vi "BP_outputLayer.vi"(0 "Target_outX":dbl[](array[numeric]), 1 "Out_hx":dbl[](array[numeric]), 2 "Out_outX":dbl[](array[numeric]), 3 "Learning rate":dbl, 4 "Weights_outX_IN":dbl[][](array[numeric])) -> (5 "Weights_outX_OUT":dbl[][](array[numeric]))   [LabVIEW 2016]
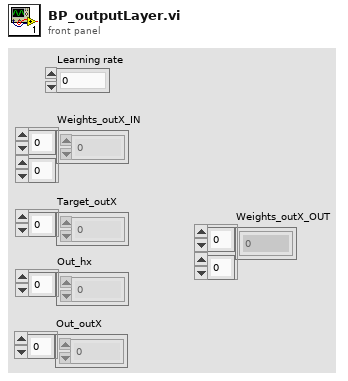
[diagram p1: front panel]
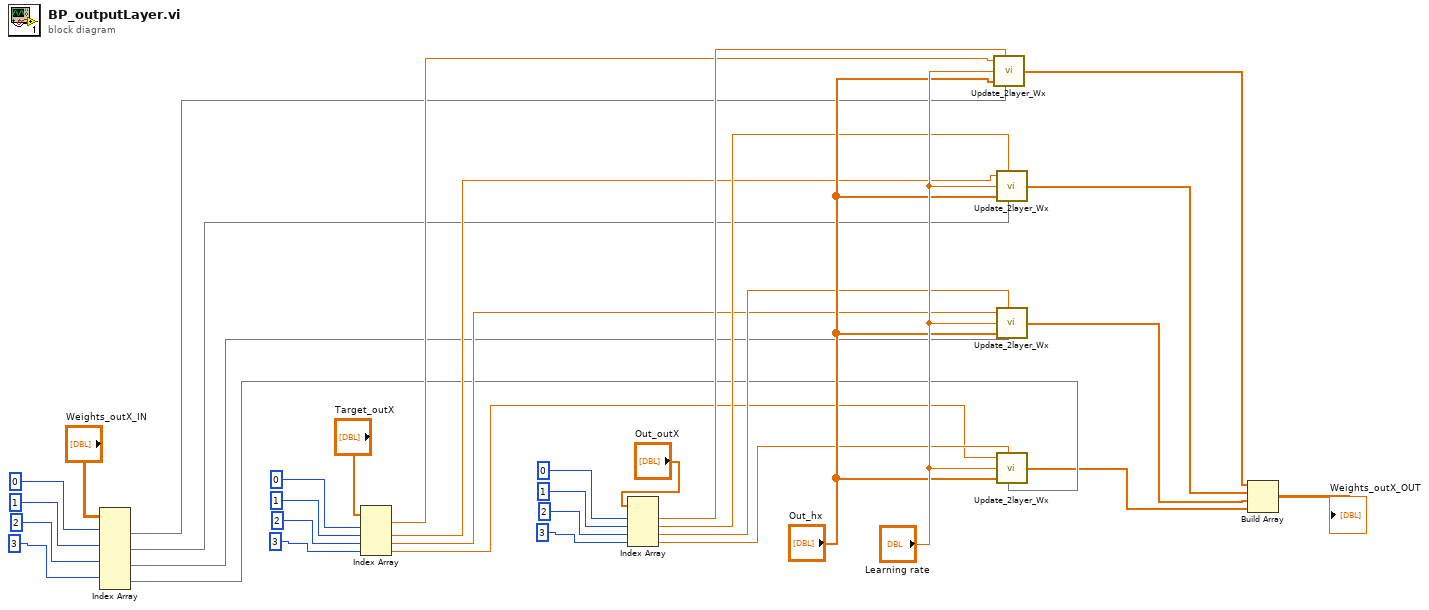
[diagram p0: block diagram]
diagram:
  n1 = Index Array(array="Weights_outX_IN", index (row) #1=0 ("index"), index (row) #2=1 ("index"), index (row) #3=2 ("index"), index (row) #4=3 ("index")) -> (element #1=w9:dbl[], element #2=w8:dbl[], element #3=w7:dbl[], element #4=w6:dbl[])  [unwired: 4 in]
  n2 = Index Array(array="Target_outX", index #1=0 ("index"), index #2=1 ("index"), index #3=2 ("index"), index #4=3 ("index")) -> (element #1=w18:dbl, element #2=w17:dbl, element #3=w16:dbl, element #4=w15:dbl)
  n3 = Index Array(array="Out_outX", index #1=0 ("index"), index #2=1 ("index"), index #3=2 ("index"), index #4=3 ("index")) -> (element #1=w27:dbl, element #2=w26:dbl, element #3=w25:dbl, element #4=w24:dbl)
  n4 = call "Update_2layer_Wx.vi"("Target_OutX"=w18, "2layer_OutX 2"=w27, "Learning rate"="Learning rate", "Array_Out_hx"="Out_hx", "Weights_2layer"=w9) -> ("Weights_2layer_updated"=w5:dbl[])
  n5 = call "Update_2layer_Wx.vi"("Target_OutX"=w17, "2layer_OutX 2"=w26, "Learning rate"="Learning rate", "Array_Out_hx"="Out_hx", "Weights_2layer"=w8) -> ("Weights_2layer_updated"=w4:dbl[])
  n6 = call "Update_2layer_Wx.vi"("Target_OutX"=w16, "2layer_OutX 2"=w25, "Learning rate"="Learning rate", "Array_Out_hx"="Out_hx", "Weights_2layer"=w7) -> ("Weights_2layer_updated"=w3:dbl[])
  n7 = call "Update_2layer_Wx.vi"("Target_OutX"=w15, "2layer_OutX 2"=w24, "Learning rate"="Learning rate", "Array_Out_hx"="Out_hx", "Weights_2layer"=w6) -> ("Weights_2layer_updated"=w2:dbl[])
  n8 = Build Array(w5, w4, w3, w2) -> (→"Weights_outX_OUT":dbl[][])
